vi "Construction_of_Subtrack(General)-1.vi"(4 "[IN] # of Track with\nFirst Problem Point":i32, 5 "[IN] Indexes for Jumps":i32[](array[numeric]), 6 "[IN] Index of First Pro\nblem Point Inside Track":i32, 7 "[IN] Minimal Subtrack\nLength for Making Desicion":i32, 8 "error IN":errorcluster, 9 "[IN] Count of variants":i32, 10 "[IN] Subtracks":T1(array[cluster]), 11 "[IN] Still connected\ntracks in group":T2) -> (0 "error OUT":errorcluster, 2 "[OUT] Subtracks":T1(array[cluster]))   [LabVIEW 2013]
doc: "The subVI builds the subtrack utilizing the previously defined array of jumps (origin, 1st, 2nd and 3rd problem points)"
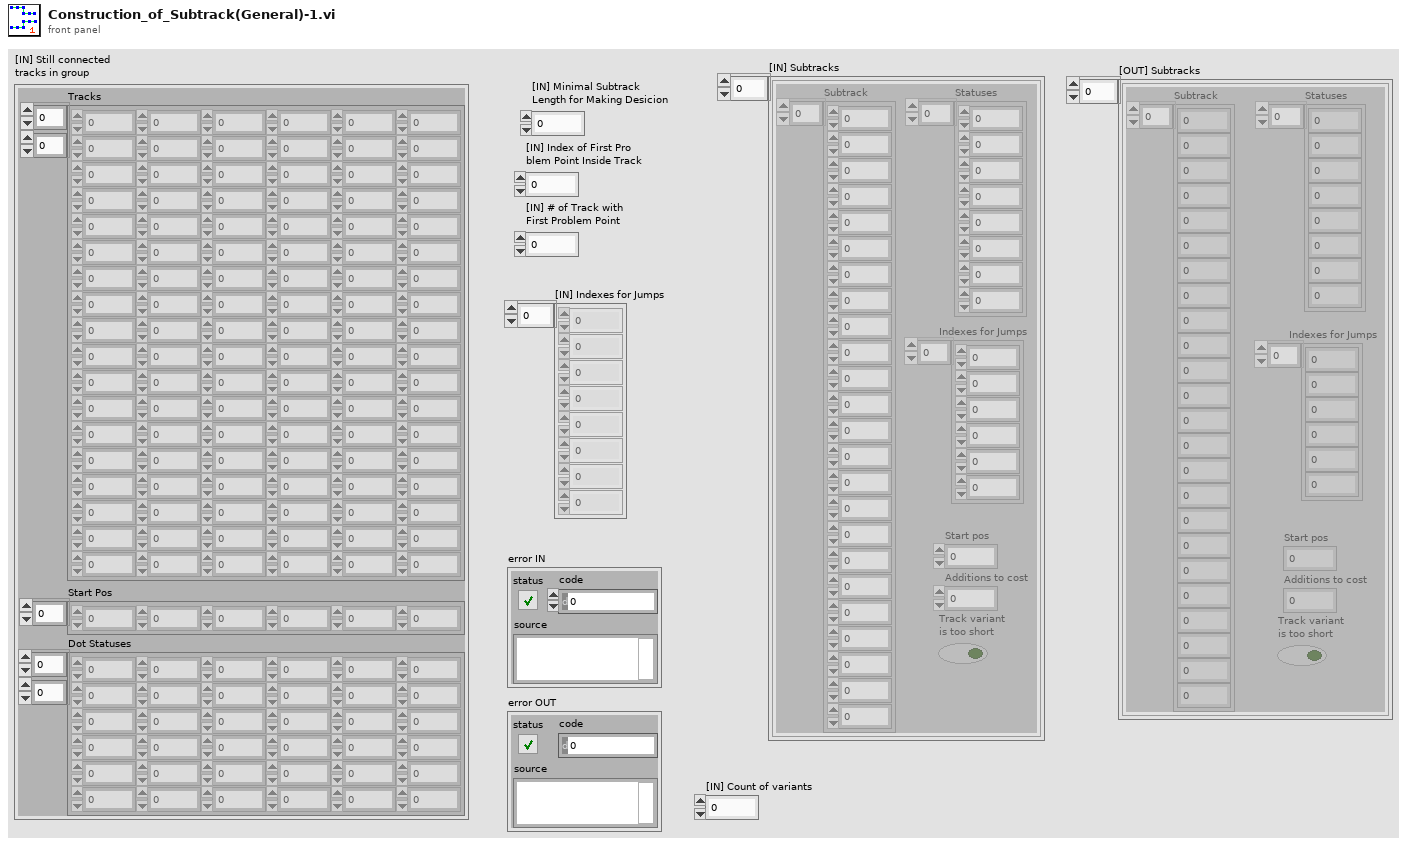
[diagram p1: front panel]
types:
  T1 = cluster{"Subtrack":dbl[], "Statuses":i16[], "Start pos":i32, "Additions to cost":i32, "Track variant \nis too short":bool, "Indexes for Jumps":i32[]}[]
  T2 = cluster{"Tracks":dbl[][], "Start Pos":i32[], "Dot Statuses":i16[][]}
  T3 = cluster{"Subtrack":dbl[], "Statuses":i16[], "Start pos":i32, "Additions to cost":i32, "Track variant \nis too short":bool, "Indexes for Jumps":i32[]}
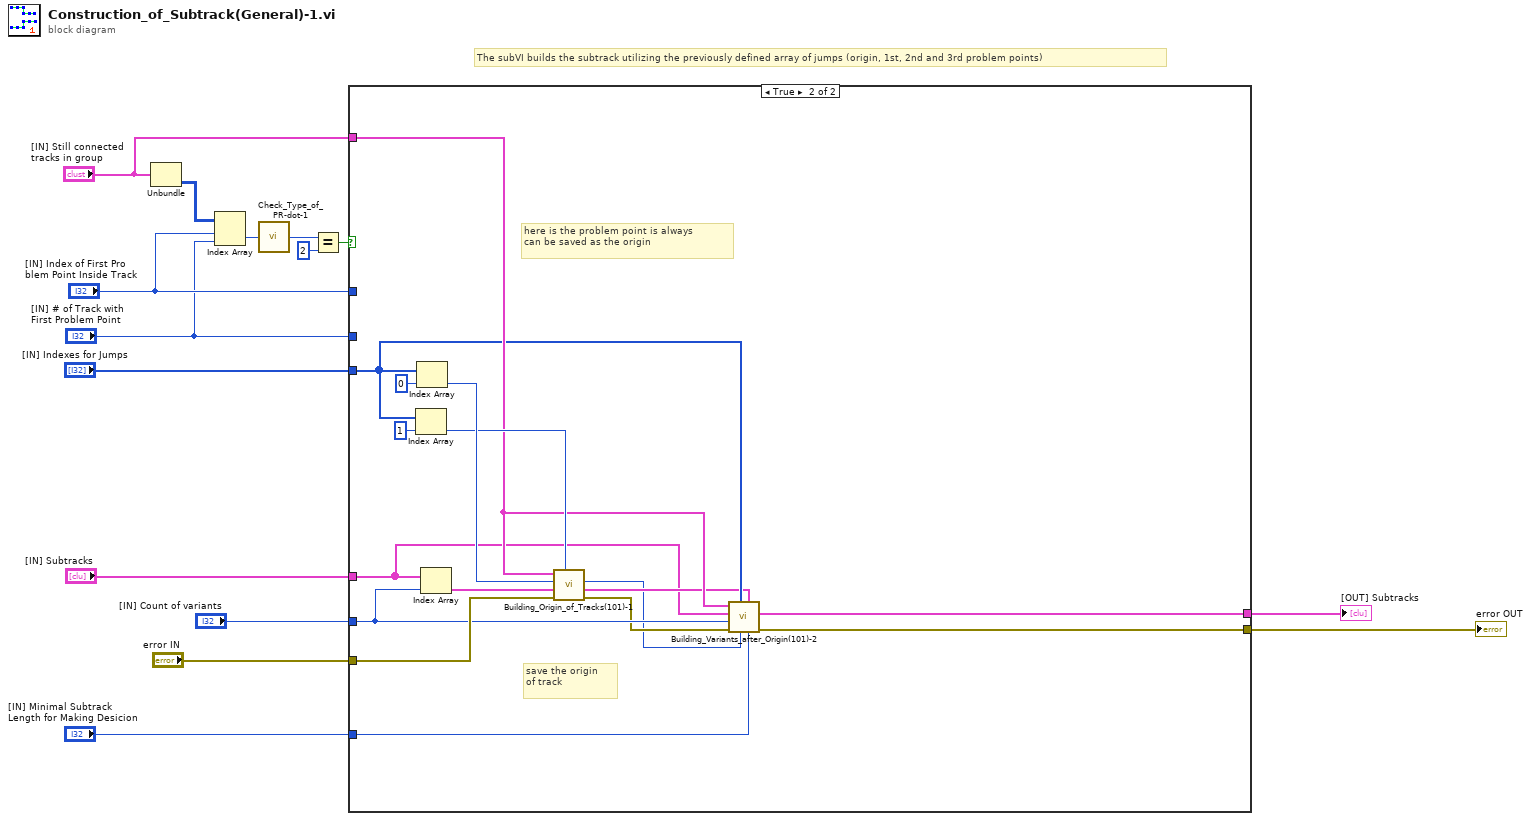
[diagram p0: block diagram]
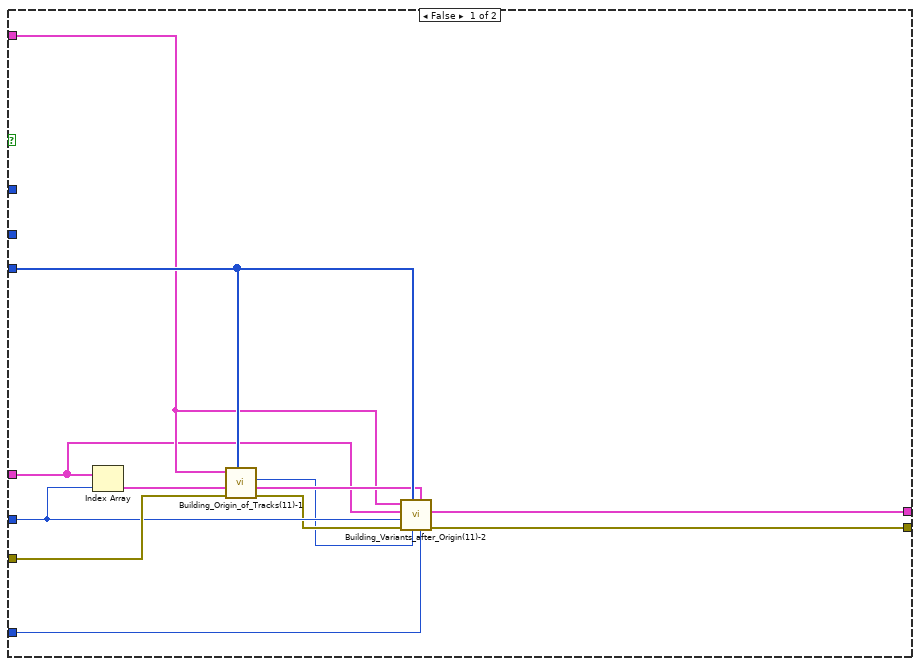
[diagram p2: hidden frame]
diagram:
  # "The subVI builds the subtrack utilizing the previously defined array of jumps (origin, 1st, 2nd and 3rd problem points)"
  n1 = Unbundle("[IN] Still connected\ntracks in group") -> ("Dot Statuses"=w5:i16[][])  [unwired: 2 out]
  n2 = Index Array(array=w5, index (row)="[IN] Index of First Pro\nblem Point Inside Track", index (col)="[IN] # of Track with\nFirst Problem Point") -> (element=w15:i16)
  n3 = call "Check_Type_of_PR-dot-1.vi"("[IN] dot status"=w15) -> ("[OUT] Type of\nproblem dot"=w13:i32)
  n4 = Equal?(x=w13, y=2) -> (x = y?=w12:bool)
  n5 = case shown="True" w12 {
    tunnel: "[IN] Index of First Pro\nblem Point Inside Track" -> [_ _]
    tunnel: "[IN] Indexes for Jumps" -> [w25 w36]
    tunnel: "[IN] Subtracks" -> [w22 w34]
    tunnel: "[IN] # of Track with\nFirst Problem Point" -> [_ _]
    tunnel: "[IN] Count of variants" -> [w21 w33]
    tunnel: "error IN" -> [w26 w40]
    tunnel: "[IN] Still connected\ntracks in group" -> [w23 w37]
    tunnel: "[IN] Minimal Subtrack\nLength for Making Desicion" -> [w18 w30]
    tunnel: [w17 w29] -> w2
    tunnel: [w16 w28] -> w1
    frame False {
      n6 = Index Array(array=w22, index=w21) -> (element=w27:T3)
      n7 = call "Building_Origin_of_Tracks(11)-1.vi"("[IN] Indexes \nfor Jumps"=w25, "error IN"=w26, "[IN] Subtrack"=w27, "[IN] Still connected\ntracks in group"=w23) -> ("error OUT"=w20:errorcluster, "[OUT] Subtrack"=w24:T3, "[OUT] Last point in subtrack"=w19:i32)  [unwired: 2 in]
      n8 = call "Building_Variants_after_Origin(11)-2.vi"("[IN] Minimal Subtrack Length"=w18, "[IN] Subtrack"=w24, "[IN] Index in the Subtrack"=w19, "[IN] Indexes for Jumps"=w25, "error IN"=w20, "[IN] Count of variants"=w21, "[IN] Subtracks"=w22, "[IN] Still connected\ntracks in group"=w23) -> ("error OUT"=w16:errorcluster, "[OUT] Subtracks"=w17:T1)  [unwired: 1 in, 1 out]
    }
    frame True {
      # "save the origin \nof track"
      # "here is the problem point is always \ncan be saved as the origin"
      n9 = Index Array(array=w36, index=1) -> (element=w38:i32)
      n10 = Index Array(array=w36, index=0) -> (element=w39:i32)
      n11 = Index Array(array=w34, index=w33) -> (element=w41:T3)
      n12 = call "Building_Origin_of_Tracks(101)-1.vi"("[IN] # part of \norigin track"=w38, "error IN"=w40, "[IN] Subtrack"=w41, "[IN] Problem point \nin the origin"=w39, "[IN] Still connected\ntracks in group"=w37) -> ("error OUT"=w32:errorcluster, "[OUT] Subtrack"=w35:T3, "[OUT] Last point in subtrack"=w31:i32)  [unwired: 1 in]
      n13 = call "Building_Variants_after_Origin(101)-2.vi"("[IN] Minimal Subtrack Length"=w30, "[IN] Subtrack"=w35, "[IN] Index in the Subtrack"=w31, "[IN] Indexes for Jumps"=w36, "error IN"=w32, "[IN] Count of variants"=w33, "[IN] Subtracks"=w34, "[IN] Still connected\ntracks in group"=w37) -> ("error OUT"=w28:errorcluster, "[OUT] Subtracks"=w29:T1)  [unwired: 1 in, 1 out]
    }
  }
  "error OUT" <- w1
  "[OUT] Subtracks" <- w2
